vi "SSH Open.vi"(8 "Error In":errorcluster, 11 "Credentials":T1) -> (0 "Error Out":errorcluster, 2 "Connected?":bool, 3 "SSH Session":refnum<k1>)   [LabVIEW 2020, in "LMH-LINX.lvlib"]
uses:
  LMH-LINX.lvlib
  C:/Users/rkalbermatter/Projects/LabVIEW Hobbyist/LINX/LabVIEW/vi.lib/MakerHub/LINX/Resources/Renci.SshNet.dll
  Resources/Renci.SshNet.dll
  SSH Unix Session Op.ctl
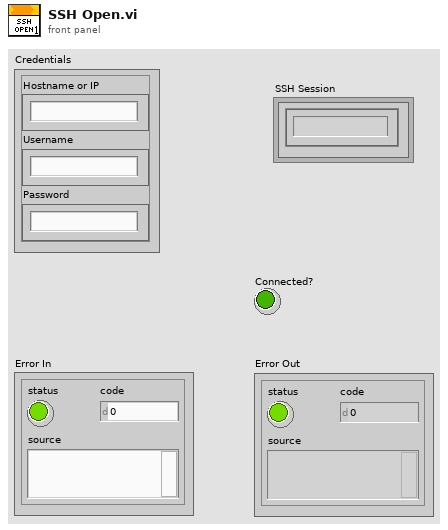
[diagram p1: front panel]
types:
  T1 = cluster{"Hostname or IP":string, "Username":string, "Password":string}
  T2 = typedef "LMH-LINX.lvlib/SSH Unix Session Op.ctl" = enum16{"New", "Get", "Delete"}
  T3 = cluster{"process ID":i32, "read file descriptor":i32, "write file descriptor":i32, "error file descriptor":i32}
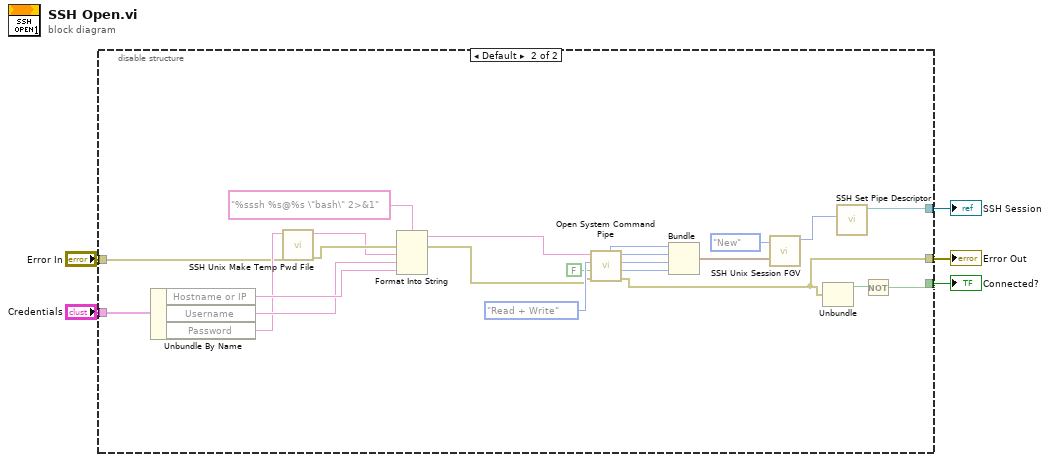
[diagram p0: block diagram]
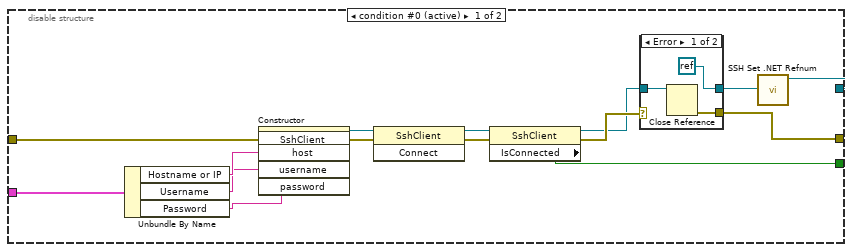
[diagram p2: hidden frame]
diagram:
  n1 = disable-structure shown="Default" {
    disable-tunnel: "Error In" -> [w16 w32]
    disable-tunnel: [w15 w26] -> w4
    disable-tunnel: "Credentials" -> [w14 w48]
    disable-tunnel: [w9 w28] -> w2
    disable-tunnel: [w7 w47] -> w1
    frame condition #0 (active) {
      n2 = Unbundle By Name(w14) -> ("Hostname or IP"=w13:string, "Username"=w12:string, "Password"=w11:string)
      n3 = constructor class="SshClient"(error in=w16, "host"=w13, "username"=w12, "password"=w11) -> (reference out=w17:refnum<k24>, error out=w18:errorcluster)  [unwired: 2 in, 4 out]
      n4 = invoke class="SshClient" method="Connect"(reference=w17, error in=w18) -> (reference out=w20:refnum<k24>, error out=w19:errorcluster)  [unwired: 1 in, 1 out]
      n5 = property class="SshClient"(reference=w20, error in=w19) -> (reference out=w8:refnum<k24>, error out=w10:errorcluster, "IsConnected"=w15:bool)
      n6 = case shown="Error" w10 {
        selector: w10 -> [_ w24]
        tunnel: [w21 w24] -> w9
        tunnel: [refnum<k0> refnum w25] -> w6
        tunnel: w8 -> [w22 w25]
        frame Error {
          n7 = Close Reference(reference=w22) -> (error out=w21:errorcluster)  [unwired: 1 in]
        }
        frame No Error {
        }
      }
      n8 = call "SSH Set .NET Refnum.vi"("SSH .NET Refnum"=w6) -> ("SSH Session"=w7:refnum<k1>)  [unwired: 9 in, 1 out]
    }
    frame condition #1 {
      n9 = Unbundle By Name(w48) -> ("Hostname or IP"=w46:string, "Username"=w43:string, "Password"=w33:string)
      n10 = call "SSH Unix Make Temp Pwd File.vi"("error in (no error)"=w32, "Password"=w33) -> ("error out"=w31:errorcluster, "sshpass command prefix"=w30:string)  [unwired: 8 in]
      n11 = Format Into String(format string="%sssh %s@%s \"bash\" 2>&1", error in=w31, w30, w43, w46) -> (resulting string=w44:string, error out=w29:errorcluster)  [unwired: 1 in]
      n12 = call <vilib>:"Open System Command Pipe.vi"("command line"=w44, "mode"=enum8{"Read", "Write", "Read + Write"}."Read + Write", "return standard error fd?"=FALSE, "error in (no error)"=w29) -> ("process ID"=w40:i32, "read file descriptor"=w39:i32, "write file descriptor"=w34:i32, "error file descriptor"=w38:i32, "error out"=w28:errorcluster)
      n13 = Bundle("process ID"=w40, "read file descriptor"=w39, "write file descriptor"=w34, "error file descriptor"=w38) -> (w37:T3)  [unwired: 1 in]
      n14 = call "SSH Unix Session FGV.vi"("info in"=w37, "Operation"=SSH_Unix_Session_Op."New") -> ("Session Out"=w35:i32)  [unwired: 8 in, 1 out]
      n15 = Unbundle(w28) -> ("status"=w27:bool)  [unwired: 2 out]
      n16 = call "SSH Set Pipe Descriptor.vi"("SSH Pipe Descriptor"=w35) -> ("SSH Session"=w47:refnum<k1>)  [unwired: 9 in, 1 out]
      n17 = Not(x=w27) -> (.not. x?=w26:bool)
    }
  }
  "Error Out" <- w2
  "SSH Session" <- w1
  "Connected?" <- w4
